vi "ultrasonic_filtering.vi"() -> ()   [LabVIEW 2023]
uses:
  <vilib>/MakerHub/LINX/Private/Device/Type Defs/Stimulus Pulse.ctl
  <vilib>/MakerHub/LINX/Public/Utilities/Open Serial.vi
  <vilib>/measure/maspectr.llb/FFT Power Spectrum and PSD for 1 Chan.vi
  <vilib>/MakerHub/LINX/LMH-LINX.lvlib
  <vilib>/MakerHub/LINX/Public/Sensors/Distance/Ultrasonic/Ultrasonic.lvlib
  <vilib>/measure/NI_MABase.lvlib
  <vilib>/measure/NI_MAPro.lvlib
  <vilib>/MakerHub/LINX/Private/Device/Device.lvlib
panel:
  in  "standard diviation":dbl=0.01 caption="Numeric" min=0.0001 max=0.01 format="%#_6f"
  out "?":u32
  out "?":u8(slide) scale=0.0..100.0
  out "?":u8(slide) scale=0.0..100.0
  out "?":dbl format="%#_2p"
  out "filtered wave but still not smooth":dynamicdata(graph)
  out "PSD of wave with noise removed":cluster{"f0":dbl, "df":dbl, "magnitude":dbl[]}(graph)
  out "orginal wave + gaussian (noisy wave)":waveform(dbl)(graph)
  out "?":dbl format="%#_2p"
  out "final wave":dynamicdata(graph)
  out "origenal wave":dbl(graph)
  in  "stop":bool
  in  "?":u32(colorbox)
  # "Centimeters"
  # "Centimeters after filtering"
  # "Centimeters after filtering"
  # "Centimeters"
  # "pulse time (uS)"
  # "standard deviation"
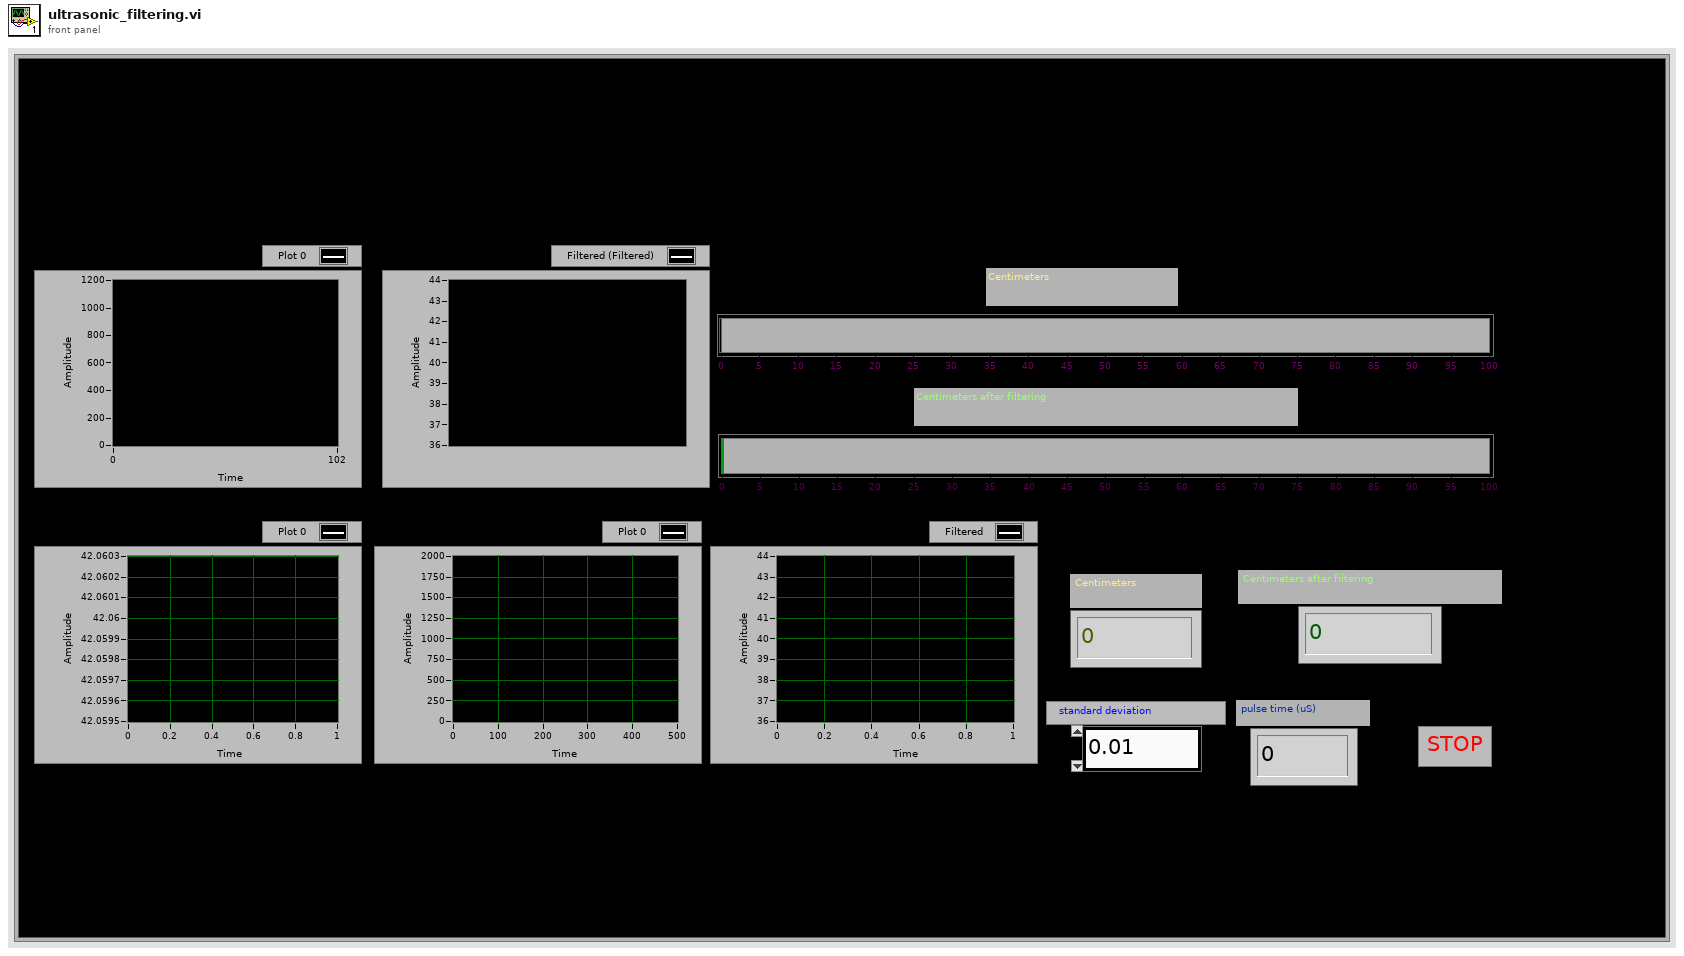
[diagram p1: front panel]
types:
  T1 = typedef "LMH-LINX.lvlib/LINX Ref.ctl" = cluster{"IO":T2, "Interface":T3, "LINX Device Config":T4}
  T2 = typedef "LMH-LINX.lvlib/Platform.ctl" = enum16{"Remote", "Local"}
  T3 = typedef "LMH-LINX.lvlib/Interface.ctl" = enum16{"Serial", "TCP"}
  T4 = typedef "LMH-LINX.lvlib/Device.lvlib/LINX Device Config.ctl" = cluster{"Interface":T3, "COM Port":refnum<visa-resource-name>, "TCP Configuration":T5, "Device Family":u8, "Device ID":u8, "Device Name":string, "TCP Ref":refnum<k5>, "Channels":T6}
  T5 = typedef "LMH-LINX.lvlib/Device.lvlib/TCP Config.ctl" = cluster{"IP Address":string, "Port":u16}
  T6 = typedef "LMH-LINX.lvlib/Channels.ctl" = cluster{"DI":u8[], "DO":u8[], "AI":u8[], "AO":u8[], "PWM":u8[], "QE":u8[], "UART":u8[], "I2C 2":u8[], "SPI":u8[], "CAN":u8[], "Servo":u8[], "AI Ref (V)":dbl, "AI Resolution (Bits)":u8, "AO Ref (V)":dbl, "AO Resolution (Bits)":u8}
  T7 = typedef "LMH-LINX.lvlib/Device.lvlib/Stimulus Pulse.ctl" = enum16{"None", "Active Low", "Active High"}
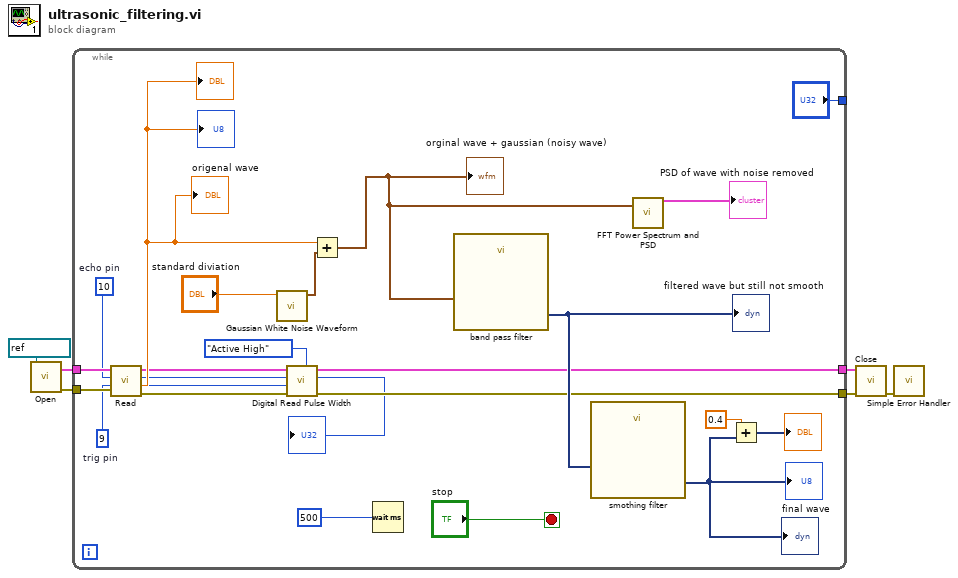
[diagram p0: block diagram]
diagram:
  n1 = call-poly <vilib>:"Open.vi"("Serial Port"=refnum<visa-resource-name> "COM3") -> ("Error Out"=w4:errorcluster, "LINX Resource"=w6:T1)  [unwired: 8 in, 1 out]
  n2 = while {
    tunnel: w6 -> [w28]
    tunnel: [w19] -> w5
    tunnel: w4 -> [w27]
    tunnel: [w17] -> w3
    tunnel: ["?"] -> _
    stop <- "stop" stop-if-true
    w15 = u8 10  # echo pin
    w10 = u8 9  # trig pin
    n3 = call <vilib>:"Read.vi"("Error In"=w27, "DO Channel"=w10, "DI Channel"=w15, "LINX Resource"=w28) -> ("Error Out"=w18:errorcluster, "Centimeters"=w21:dbl, "LINX Resource"=w20:T1)  [unwired: 4 in, 1 out]
    "origenal wave" <- w21
    "?" <- w21
    "?" <- w21
    n4 = call <vilib>:"Gaussian White Noise Waveform.vi"("standard deviation"="standard diviation") -> ("signal out"=w24:waveform(dbl))  [unwired: 9 in, 1 out]
    n5 = call <vilib>:"Digital Read Pulse Width.vi"("Stimulus Pulse (Active High)"=Stimulus_Pulse."Active High", "Error In"=w18, "DO Channel"=w10, "DI Channel"=w15, "LINX Resource"=w20) -> ("Error Out"=w17:errorcluster, "Pulse Width (uS)"=→"?":u32, "LINX Resource"=w19:T1)  [unwired: 4 in]
    n6 = Add(x=w21, y=w24) -> (x+y=w11:waveform(dbl))
    "orginal wave + gaussian (noisy wave)" <- w11
    n7 = Wait (ms)(milliseconds to wait=u32 500) -> ()  [unwired: 1 out]
    n8 = call "band pass filter"("Signal"=w11) -> ("Filtered Signal"=w22:dynamicdata)  [unwired: 9 in, 1 out]
    "filtered wave but still not smooth" <- w22
    n9 = call "smothing filter"("Signal"=w22) -> ("Filtered Signal"=w9:dynamicdata)  [unwired: 9 in, 1 out]
    "final wave" <- w9
    "?" <- w9
    n10 = call-poly <vilib>:"FFT Power Spectrum and PSD.vi"("time signal"=w11) -> ("Power Spectrum / PSD"=→"PSD of wave with noise removed":cluster{"f0":dbl, "df":dbl, "magnitude":dbl[]})  [unwired: 7 in, 3 out]
    n11 = Add(x=0.4, y=w9) -> (x+y=→"?":dynamicdata)
  }
  n12 = call <vilib>:"Close.vi"("Error In"=w3, "LINX Resource"=w5) -> ("Error Out"=w1:errorcluster)  [unwired: 9 in]
  n13 = call <vilib>:"Simple Error Handler.vi"("error in (no error)"=w1) -> ()  [unwired: 4 in, 5 out]
